vi "PID_auto.vi"(10 "vitesse voulu":dbl format="%#_13g") -> ()   [LabVIEW 2015]
uses:
  <vilib>/addons/control/pid/pid.llb/PID (DBL).vi
  <vilib>/addons/control/pid/NI_PID_pid.lvlib
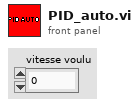
[diagram p1: front panel]
types:
  T1 = cluster{"proportional gain (Kc)":dbl, "integral time (Ti, min)":dbl, "derivative time (Td, min)":dbl}
  T2 = typedef "WPI_EncoderDevRef.ctl" = cluster{"DevStatus":errorcluster, "EncoderIndex":T3, "CounterIndex":T4, "DistancePerCount":dbl, "Decoding Type":T5}
  T3 = typedef "FPGA_EncoderIdx.ctl" = enum8{"Enc 0", "Enc 1", "Enc 2", "Enc 3", "Enc 4", "Enc 5", "Enc 6", "Enc 7", "Invalid"}
  T4 = typedef "FPGA_CounterCtrSystemIndex.ctl" = enum8{"Ctr 0", "Ctr 1", "Ctr 2", "Ctr 3", "Ctr 4", "Ctr 5", "Ctr 6", "Ctr 7", "Invalid"}
  T5 = typedef "WPI_EncoderType.ctl" = enum16{"1x", "2x", "4x"}
  T6 = typedef "WPI_MotorControlDeviceRef.ctl" = cluster{"DeviceStatus":errorcluster, "Type":T7, "PWM":cluster{"PWM Channel":T8, "DeadBand":T9}, "CAN":cluster{"Device Number":u8, "Control Mode":T10, "Semaphore":T11, "Max Vout":dbl, "TalonSRX Control Mode":T12}, "Invert":bool}
  T7 = typedef "WPI_MotorControlType.ctl" = enum16{"PWM", "CAN", "CANTalonSRX"}
  T8 = typedef "FPGA_DIOPWMChannel.ctl" = enum8{"PWM 0", "PWM 1", "PWM 2", "PWM 3", "PWM 4", "PWM 5", "PWM 6", "PWM 7", "PWM 8", "PWM 9", "PWM MXP 0", "PWM MXP 1", "PWM MXP 2", "PWM MXP 3", "PWM MXP 4", "PWM MXP 5", "PWM MXP 6", "PWM MXP 7", "PWM MXP 8", "PWM MXP 9", "Invalid"}
  T9 = typedef "WPI_PWMDeadband.ctl" = cluster{"Name":string, "maxPositivePwm":i32, "minPositivePwm":i32, "centerPwm":i32, "maxNegativePwm":i32, "minNegativePwm":i32, "angularRange":u16}
  T10 = typedef "WPI_CANJaguar_ControlMode.ctl" = enum8{"Percent VBus", "Current", "Speed", "Position", "Voltage"}
  T11 = typedef "Semaphore RefNum" = refnum<k1>
  T12 = typedef "WPI_CANTalonSRX_APIControlMode.ctl" = enum8{"Percent VBus", "Speed", "Position", "Slave", "Unchanged / Invalid", "Voltage Compensation", "Current", "Motion Profile"}
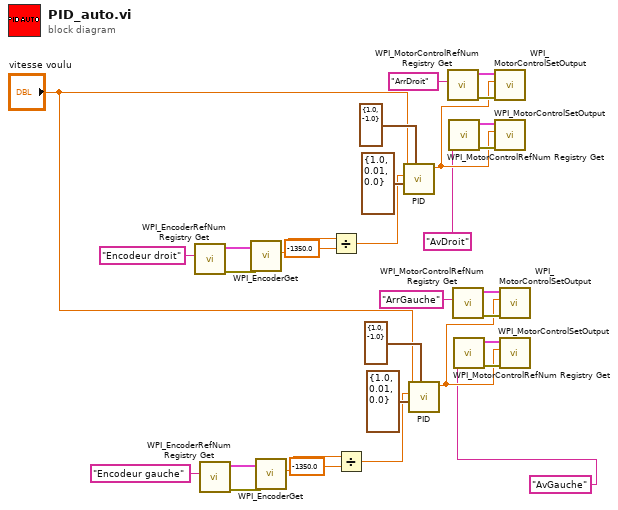
[diagram p0: block diagram]
diagram:
  n1 = call <vilib>:"WPI_EncoderRefNum Registry Get.vi"("refnum name"="Encodeur droit") -> ("error out"=w29:errorcluster, "EncoderDevRef"=w28:T2)  [unwired: 9 in]
  n2 = call <vilib>:"WPI_EncoderRefNum Registry Get.vi"("refnum name"="Encodeur gauche") -> ("error out"=w14:errorcluster, "EncoderDevRef"=w13:T2)  [unwired: 9 in]
  n3 = call <vilib>:"WPI_EncoderGet.vi"("error in (no error)"=w29, "EncoderDevRef"=w28) -> ("Distance"=w27:dbl)  [unwired: 4 in, 5 out]
  n4 = call <vilib>:"WPI_EncoderGet.vi"("error in (no error)"=w14, "EncoderDevRef"=w13) -> ("Distance"=w12:dbl)  [unwired: 4 in, 5 out]
  n5 = Divide(x=w27, y=-1350.0) -> (x/y=w25:dbl)
  n6 = Divide(x=w12, y=-1350.0) -> (x/y=w10:dbl)
  n7 = call-poly <vilib>:"PID.vi"("output range"=cluster{"output high":dbl, "output low":dbl} {"output high"=1.0, "output low"=-1.0}, "PID gains"=T1 {"proportional gain (Kc)"=1.0, "integral time (Ti, min)"=0.01, "derivative time (Td, min)"=0.0}, "process variable"=w25, "setpoint"="vitesse voulu") -> ("output"=w20:dbl)  [unwired: 6 in, 1 out]
  n8 = call-poly <vilib>:"PID.vi"("output range"=cluster{"output high":dbl, "output low":dbl} {"output high"=1.0, "output low"=-1.0}, "PID gains"=T1 {"proportional gain (Kc)"=1.0, "integral time (Ti, min)"=0.01, "derivative time (Td, min)"=0.0}, "process variable"=w10, "setpoint"="vitesse voulu") -> ("output"=w5:dbl)  [unwired: 6 in, 1 out]
  n9 = call <vilib>:"WPI_MotorControlRefNum Registry Get.vi"("refnum name"="ArrDroit") -> ("error out"=w22:errorcluster, "MotorControlDevRef"=w21:T6)  [unwired: 9 in]
  n10 = call <vilib>:"WPI_MotorControlRefNum Registry Get.vi"("refnum name"="AvDroit") -> ("error out"=w24:errorcluster, "MotorControlDevRef"=w23:T6)  [unwired: 9 in]
  n11 = call <vilib>:"WPI_MotorControlRefNum Registry Get.vi"("refnum name"="ArrGauche") -> ("error out"=w7:errorcluster, "MotorControlDevRef"=w6:T6)  [unwired: 9 in]
  n12 = call <vilib>:"WPI_MotorControlRefNum Registry Get.vi"("refnum name"="AvGauche") -> ("error out"=w9:errorcluster, "MotorControlDevRef"=w8:T6)  [unwired: 9 in]
  n13 = call <vilib>:"WPI_MotorControlSetOutput.vi"("error in (no error)"=w22, "Output"=w20, "MotorControlDevRef"=w21) -> ()  [unwired: 6 in, 3 out]
  n14 = call <vilib>:"WPI_MotorControlSetOutput.vi"("error in (no error)"=w24, "Output"=w20, "MotorControlDevRef"=w23) -> ()  [unwired: 6 in, 3 out]
  n15 = call <vilib>:"WPI_MotorControlSetOutput.vi"("error in (no error)"=w7, "Output"=w5, "MotorControlDevRef"=w6) -> ()  [unwired: 6 in, 3 out]
  n16 = call <vilib>:"WPI_MotorControlSetOutput.vi"("error in (no error)"=w9, "Output"=w5, "MotorControlDevRef"=w8) -> ()  [unwired: 6 in, 3 out]
